vi "main.vi"() -> ()   [LabVIEW 2017]
panel:
  out "a+b+c+d":dbl
  in  "d":dbl
  out "a+b+c":dbl
  in  "c":dbl
  out "a+b":dbl
  in  "b":dbl
  in  "a":dbl
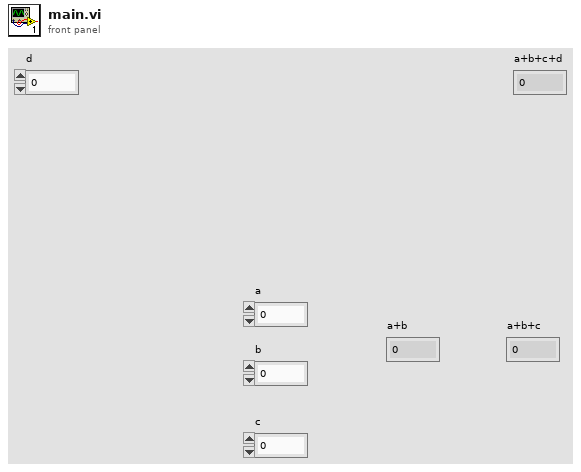
[diagram p1: front panel]
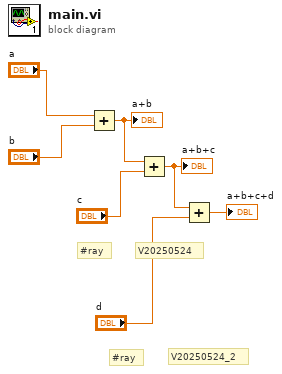
[diagram p0: block diagram]
diagram:
  # "V20250524_2"
  # "#ray"
  # "V20250524"
  # "#ray"
  n1 = Add(x="a", y="b") -> (x+y=w5:dbl)
  "a+b" <- w5
  n2 = Add(x=w5, y="c") -> (x+y=w3:dbl)
  "a+b+c" <- w3
  n3 = Add(x=w3, y="d") -> (x+y=→"a+b+c+d":dbl)
